vi "Global 2.vi"() -> ()   [LabVIEW 2013]
uses:
  <vilib>/ActorFramework/Message Enqueuer/Message Enqueuer.lvclass
panel:
  out "Observer Array 2":refnum<class "Message Enqueuer.lvclass">[](array[class])
  out "i":i32
  out "error out":errorcluster
  out "size":dbl
  out "Observer Array":refnum<class "Message Enqueuer.lvclass">[](array[class])
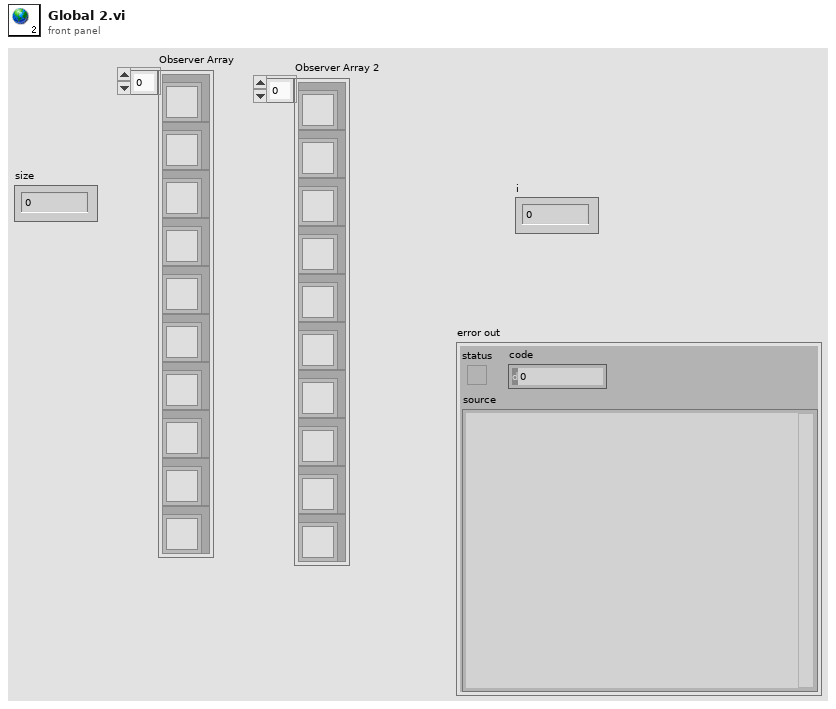
[diagram p1: front panel]
diagram:
